vi "test_Get RIO Resource.vi"(8 "error in (no error)":errorcluster, 11 "TestCase in":refnum<class "FPGA Addon Scripting API Unit Tests.lvclass">=refnum) -> (0 "error out":errorcluster, 3 "TestCase out":refnum<class "FPGA Addon Scripting API Unit Tests.lvclass">)   [LabVIEW 2026, in "FPGA Addon Scripting API Unit Tests.lvclass"]
uses:
  FPGA Addon Scripting API Unit Tests.lvclass
  FPGA Addon Test Class/FPGA Addon Test Class.lvclass
  APIs/Scripting API/Scripting API.lvlib
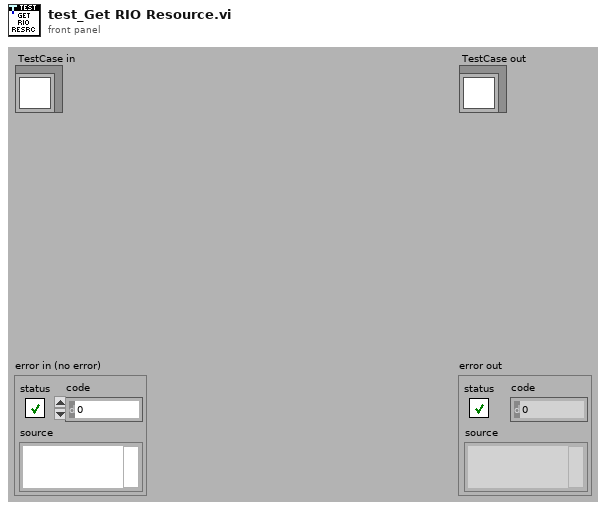
[diagram p1: front panel]
types:
  T1 = typedef "Custom Device API.lvlib/Custom Device Item Ref.ctl" = u64
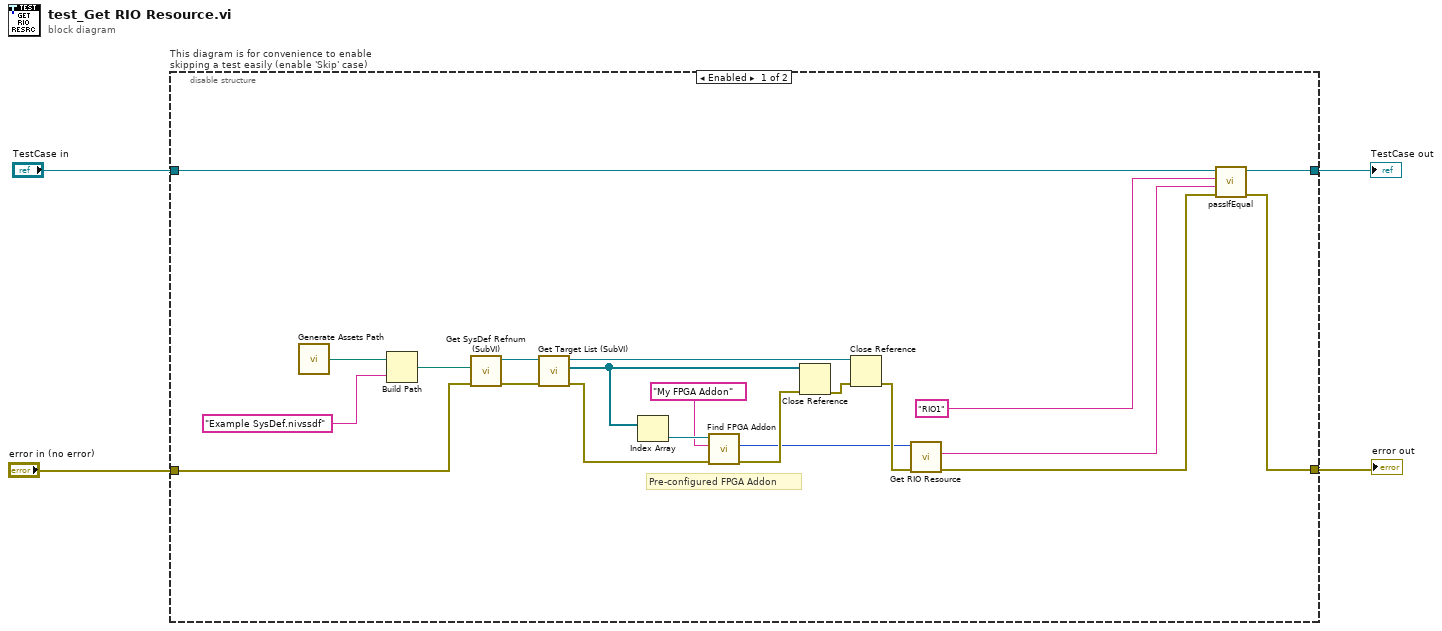
[diagram p0: block diagram]
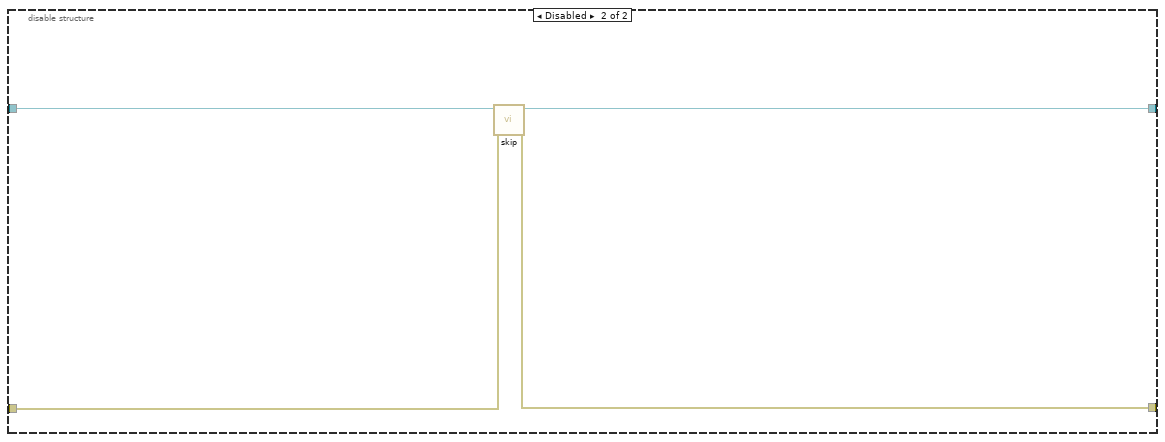
[diagram p2: hidden frame]
diagram:
  n1 = disable-structure "This diagram is for convenience to enable skipping a test easily (enable 'Skip' case)" shown="Enabled" {
    disable-tunnel: "TestCase in" -> [w12 w29]
    disable-tunnel: [w10 w27] -> w1
    disable-tunnel: [w11 w28] -> w3
    disable-tunnel: "error in (no error)" -> [w21 w26]
    frame Enabled {
      # "Pre-configured FPGA Addon"
      n2 = call "Generate Assets Path.vi"() -> ("Assets path"=w25:path)
      n3 = Build Path(base path=w25, name or relative path="Example SysDef.nivssdf") -> (appended path=w23:path)
      n4 = call "Get SysDef Refnum (SubVI).vi"("error in (no error)"=w21, "System Definition path"=w23) -> ("error out"=w20:errorcluster, "NationalInstruments.VeriStand.SystemDefinitionAPI.SystemDefinition"=w22:refnum<k39>)  [unwired: 8 in]
      n5 = call "Get Target List (SubVI).vi"("error in (no error)"=w20, "NationalInstruments.VeriStand.SystemDefinitionAPI.SystemDefinition"=w22) -> ("error out"=w15:errorcluster, "Target List Refnums"=w19:refnum<k39>[], "NationalInstruments.VeriStand.SystemDefinitionAPI.SystemDefinition"=w18:refnum<k39>)  [unwired: 7 in]
      n6 = Index Array(array=w19) -> (element=w16:refnum<k39>)  [unwired: 1 in]
      n7 = call "Find FPGA Addon.vi"("error in"=w15, "FPGA addon name"="My FPGA Addon", "NationalInstruments.VeriStand.SystemDefinitionAPI.Target"=w16) -> ("error out"=w13:errorcluster, "FPGA addon refnum out"=w8:T1)  [unwired: 5 in, 2 out]
      n8 = Close Reference(reference=w19, error in (no error)=w13) -> (error out=w17:errorcluster)
      n9 = Close Reference(reference=w18, error in (no error)=w17) -> (error out=w9:errorcluster)
      n10 = call "Get RIO Resource.vi"("error in"=w9, "FPGA addon refnum in"=w8) -> ("error out"=w7:errorcluster, "RIO resource"=w6:string)  [unwired: 7 in, 1 out]
      n11 = call-dynamic "passIfEqual.vi"("error in (no error)"=w7, "y"=w6, "x"="RIO1" ("RIO resource"), "TestCase in"=w12) -> ("error out"=w11:errorcluster, "TestCase out"=w10:refnum<class "FPGA Addon Scripting API Unit Tests.lvclass">)  [unwired: 6 in]
    }
    frame Disabled {
      # "skip test result while test is under development"
      n12 = call <vilib>:"skip.vi"("error in (no error)"=w26, "TestCase in"=w29) -> ("error out"=w28:errorcluster, "TestCase out"=w27:refnum<class "FPGA Addon Scripting API Unit Tests.lvclass">)  [unwired: 8 in]
    }
  }
  "error out" <- w3
  "TestCase out" <- w1
